vi "PS_Gaussians.vi"(3 "output control":T1, 4 "data":variant, 5 "X":dbl[](array[numeric]), 6 "a":dbl[](array[numeric])) -> (0 "error out":errorcluster, 1 "f'(X,a)":dbl[][](array[numeric]), 2 "f(X,a)":dbl[](array[numeric]))   [LabVIEW 2011]
uses:
  <vilib>/gmath/NumericalOptimization/LM_output select.ctl
  <vilib>/gmath/NI_Gmath.lvlib
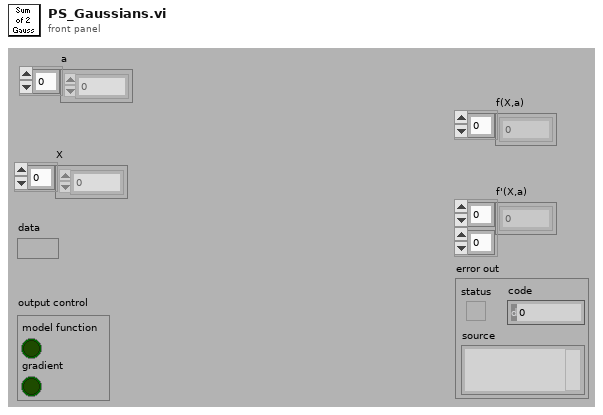
[diagram p1: front panel]
types:
  T1 = typedef "NI_Gmath.lvlib/LM_output select.ctl" = cluster{"model function":bool, "gradient":bool}
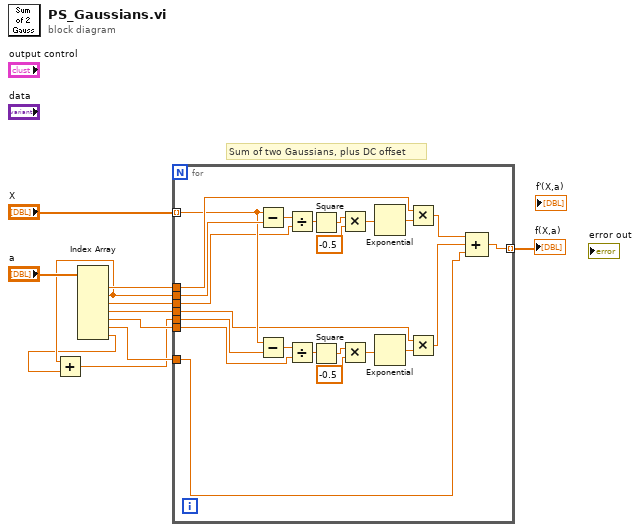
[diagram p0: block diagram]
diagram:
  # "Sum of two Gaussians, plus DC offset"
  n1 = Index Array(array="a") -> (element #1=w10:dbl, element #2=w2:dbl, element #3=w9:dbl, element #4=w8:dbl, element #5=w4:dbl, element #6=w5:dbl, element #7=w1:dbl)  [unwired: 7 in]
  n2 = Add(x=w2, y=w1) -> (x+y=w3:dbl)
  n3 = for {
    tunnel: "X" -> [w28] mode=indexing
    tunnel: w10 -> [w32]
    tunnel: w2 -> [w34]
    tunnel: w9 -> [w19]
    tunnel: w8 -> [w26]
    tunnel: w3 -> [w27]
    tunnel: w4 -> [w18]
    tunnel: w5 -> [w12]
    tunnel: [w23] -> w7 mode=indexing
    n4 = Subtract(x=w28, y=w34) -> (x-y=w20:dbl)
    n5 = Subtract(x=w28, y=w27) -> (x-y=w17:dbl)
    n6 = Divide(x=w20, y=w19) -> (x/y=w33:dbl)
    n7 = Divide(x=w17, y=w18) -> (x/y=w29:dbl)
    n8 = Square(x=w33) -> (x^2=w16:dbl)
    n9 = Square(x=w29) -> (x^2=w15:dbl)
    n10 = Multiply(x=w16, y=-0.5) -> (x*y=w22:dbl)
    n11 = Multiply(x=w15, y=-0.5) -> (x*y=w21:dbl)
    n12 = Exponential(1:w22) -> (0:w31:dbl)
    n13 = Exponential(1:w21) -> (0:w30:dbl)
    n14 = Multiply(x=w32, y=w31) -> (x*y=w25:dbl)
    n15 = Multiply(x=w26, y=w30) -> (x*y=w24:dbl)
    n16 = Compound Arithmetic op=ADD(w25, w24, w12) -> (w23:dbl)
  }
  "f(X,a)" <- w7
